vi "Accel2Pos_RatePoints.vi"(8 "Points":u32, 9 "Rate (hz)":dbl, 10 "Start (s)":dbl, 11 "Accel":T1(array[cluster])=[{"A"=5.0, "B"=11.107207345395915, "Start"=0.3585786437626905, "End"=0.6414213562373094, "Center"=0.5, "Velocity"=0.0, "Position"=0.7071067811865475}, {"A"=-5.0, "B"=5.553603672697958, "Start"=1.631370849898476, "End"=2.197056274847714, "Center"=1.914213562373095, "Velocity"=0.7071067811865475, "Position"=-0.7071067811865475}, {"A"=5.0, "B"=11.107207345395915, "Start"=3.18700576850888, "End"=3.4698484809834995, "Center"=3.32842712474619, "Velocity"=-0.7071067811865475, "Position"=0.0}]) -> (1 "Times":dbl[](array[numeric]), 2 "Velocities":dbl[](array[numeric]), 3 "Positions":dbl[](array[numeric]))   [LabVIEW 2014]
panel:
  out "Position/Velocity":cluster{cluster{dbl, dbl}[]}[](graph)
  out "EndTime":dbl
  out "EndIndex":i32
  out "StartIndex":i32
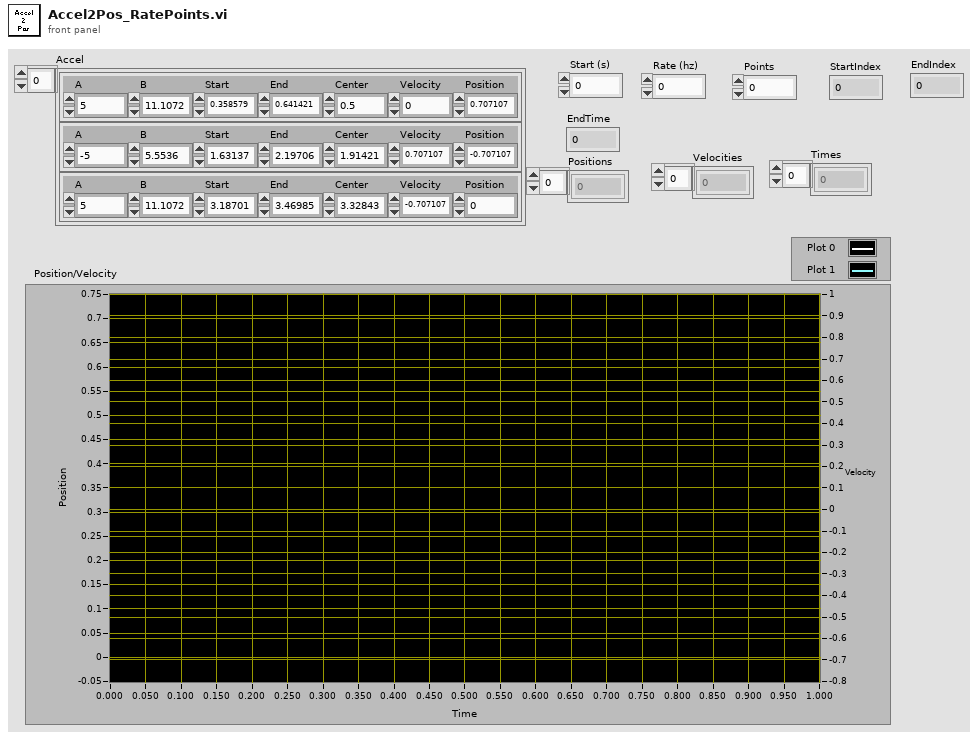
[diagram p1: front panel]
types:
  T1 = cluster{"A":dbl, "B":dbl, "Start":dbl, "End":dbl, "Center":dbl, "Velocity":dbl, "Position":dbl}[]
  T2 = cluster{"A":dbl, "B":dbl, "Start":dbl, "End":dbl, "Center":dbl, "Velocity":dbl, "Position":dbl}
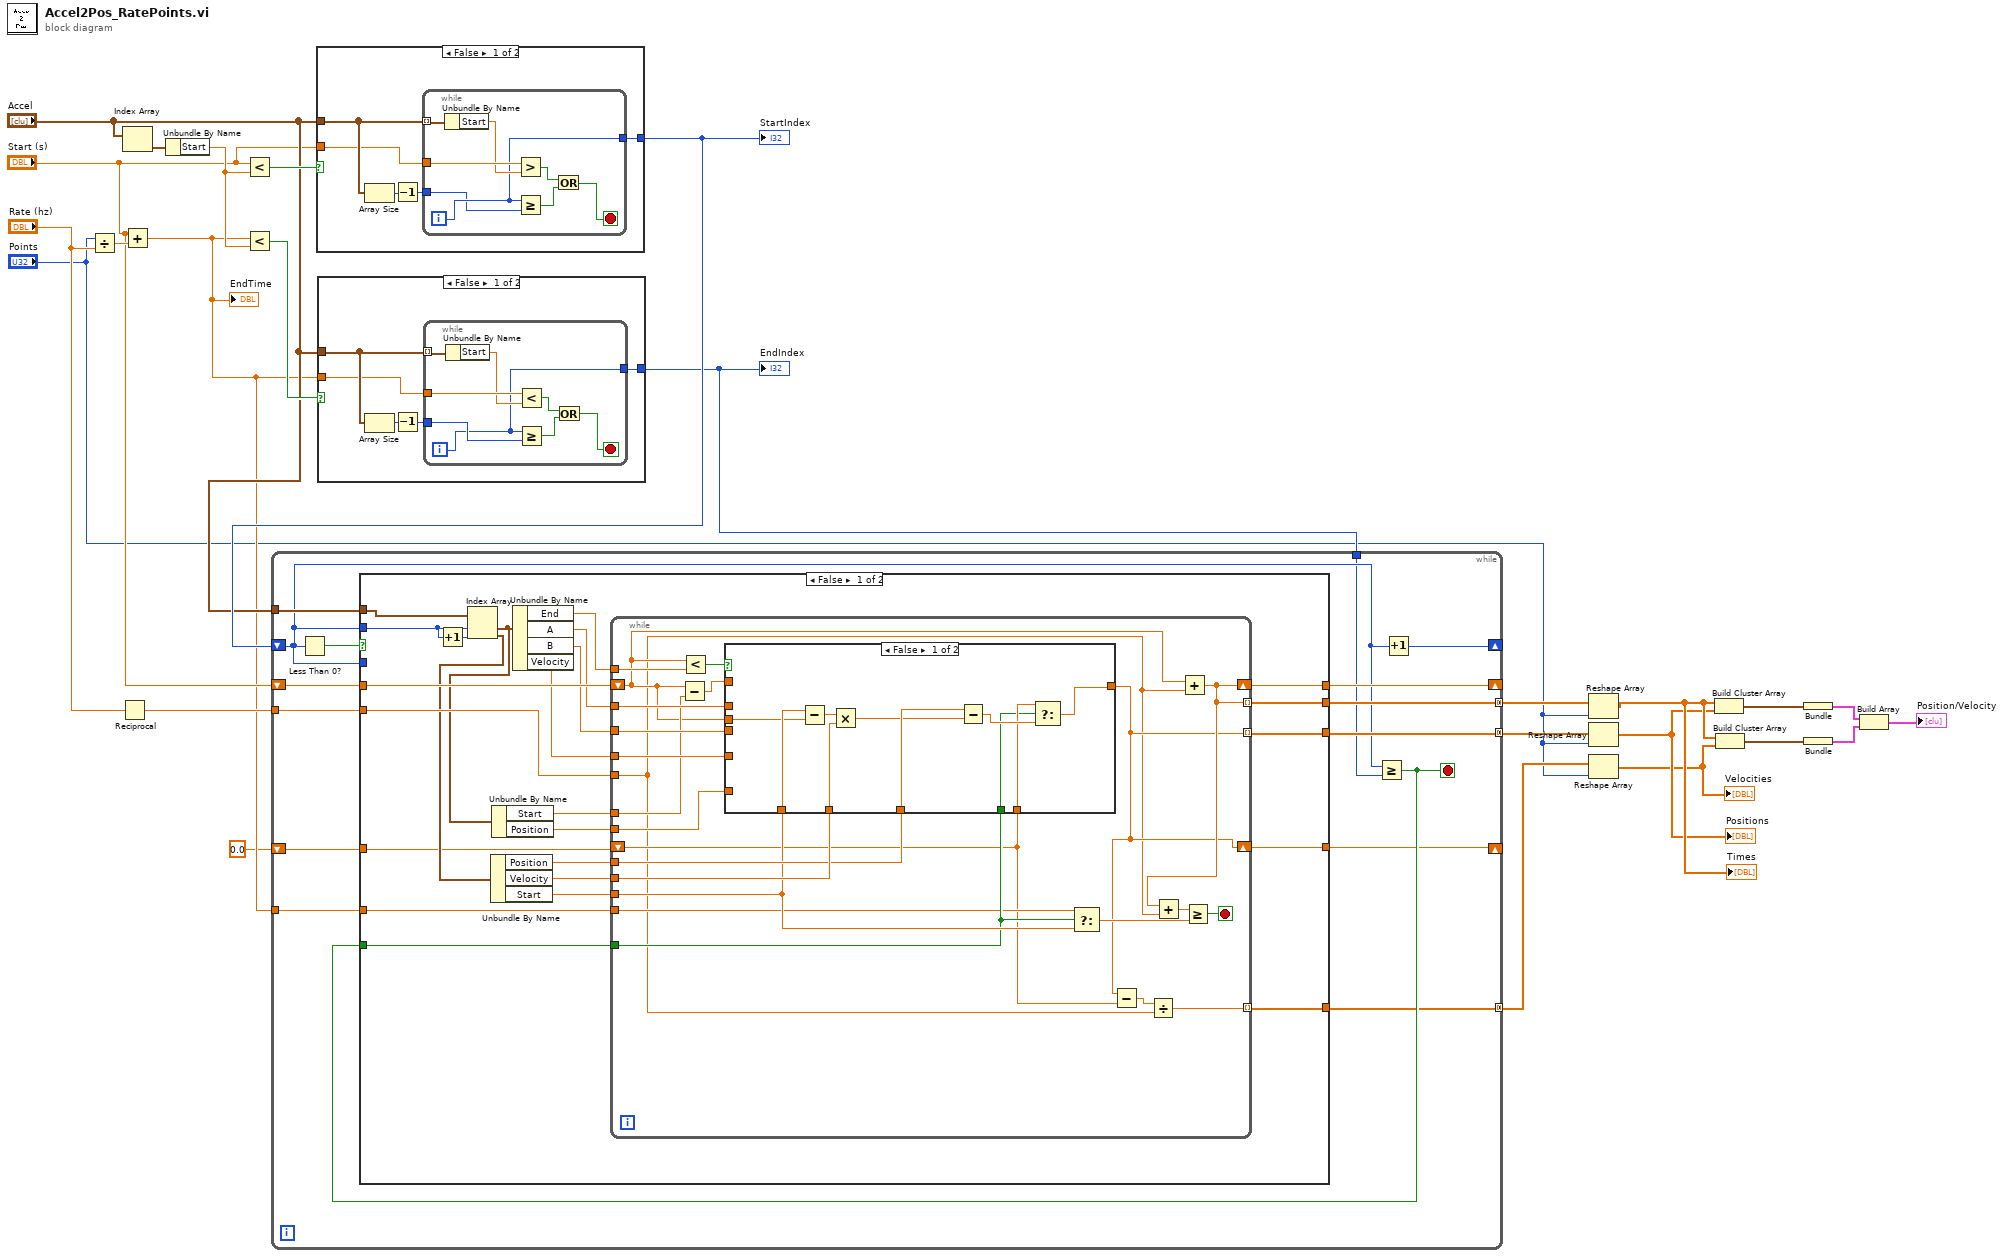
[diagram p0: block diagram]
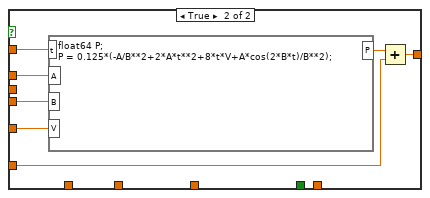
[diagram p2: hidden frame]
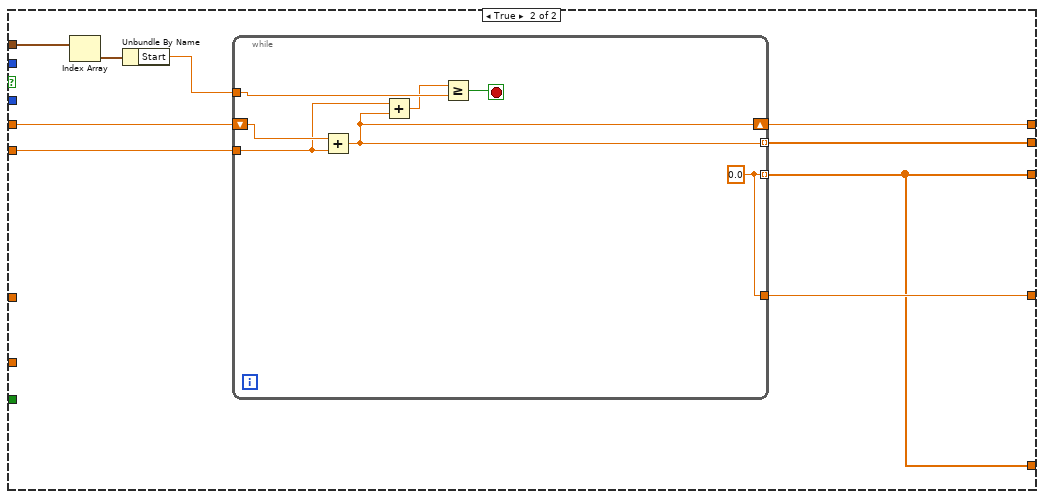
[diagram p3: hidden frame]
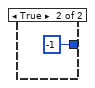
[diagram p4: hidden frame]
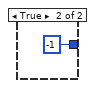
[diagram p5: hidden frame]
diagram:
  n1 = Divide(x="Points", y="Rate (hz)") -> (x/y=w21:dbl)
  n2 = Reciprocal(x="Rate (hz)") -> (1/x=w16:dbl)
  n3 = Index Array(array="Accel") -> (element=w25:T2)  [unwired: 1 in]
  n4 = Add(x="Start (s)", y=w21) -> (x+y=w14:dbl)
  "EndTime" <- w14
  n5 = Unbundle By Name(w25) -> ("Start"=w23:dbl)
  n6 = Less?(x="Start (s)", y=w23) -> (x < y?=w24:bool)
  n7 = Less?(x=w14, y=w23) -> (x < y?=w22:bool)
  n8 = case shown="False" w24 {
    tunnel: [w30 -1] -> w20
    tunnel: "Accel" -> [w29 _]
    tunnel: "Start (s)" -> [w28 _]
    frame False {
      n9 = Array Size(array=w29) -> (size(s)=w27:i32)
      n10 = Decrement(x=w27) -> (x-1=w26:i32)
      n11 = while {
        tunnel: w29 -> [w38] mode=indexing
        tunnel: w28 -> [w37]
        tunnel: [w32] -> w30
        tunnel: w26 -> [w31]
        i -> [w32]
        stop <- w33 stop-if-true
        n12 = Unbundle By Name(w38) -> ("Start"=w36:dbl)
        n13 = Greater?(x=w37, y=w36) -> (0:w35:bool)
        n14 = Greater Or Equal?(x=w32, y=w31) -> (x >= y?=w34:bool)
        n15 = Or(x=w35, y=w34) -> (x .or. y?=w33:bool)
      }
    }
    frame True {
    }
  }
  "StartIndex" <- w20
  n16 = case shown="False" w22 {
    tunnel: [w44 -1] -> w15
    tunnel: "Accel" -> [w43 _]
    tunnel: w14 -> [w42 _]
    frame False {
      n17 = Array Size(array=w43) -> (size(s)=w41:i32)
      n18 = Decrement(x=w41) -> (x-1=w40:i32)
      n19 = while {
        tunnel: w43 -> [w52] mode=indexing
        tunnel: w42 -> [w51]
        tunnel: w40 -> [w49]
        tunnel: [w45] -> w44
        i -> [w45]
        stop <- w46 stop-if-true
        n20 = Unbundle By Name(w52) -> ("Start"=w50:dbl)
        n21 = Less?(x=w51, y=w50) -> (x < y?=w48:bool)
        n22 = Greater Or Equal?(x=w45, y=w49) -> (x >= y?=w47:bool)
        n23 = Or(x=w48, y=w47) -> (x .or. y?=w46:bool)
      }
    }
    frame True {
    }
  }
  "EndIndex" <- w15
  n24 = while {
    shift-right: [w60] -> _
    shift-left: w20 -> [w59]
    tunnel: "Accel" -> [w65]
    shift-right: [w64] -> _
    shift-left: "Start (s)" -> [w67]
    tunnel: w16 -> [w66]
    tunnel: [w63] -> w7 mode=concatenating
    tunnel: [w62] -> w5 mode=concatenating
    tunnel: w15 -> [w58]
    tunnel: w14 -> [w57]
    shift-right: [w56] -> _
    shift-left: 0.0 -> [w55]
    tunnel: [w54] -> w3 mode=concatenating
    stop <- w61 stop-if-true
    n25 = Less Than 0?(x=w59) -> (x < 0?=w68:bool)
    n26 = Greater Or Equal?(x=w59, y=w58) -> (x >= y?=w61:bool)
    n27 = case shown="False" w68 {
      tunnel: w67 -> [w90 w139]
      tunnel: w66 -> [w89 w138]
      tunnel: w65 -> [w92 w141]
      tunnel: [w88 w136] -> w64
      tunnel: [w87 w135] -> w63
      tunnel: [w86 w133] -> w62
      tunnel: w59 -> [_ _]
      tunnel: w61 -> [w73 _]
      tunnel: w59 -> [w91 _]
      tunnel: w57 -> [w72 _]
      tunnel: [w71 w134] -> w56
      tunnel: w55 -> [w70 _]
      tunnel: [w69 w133] -> w54
      frame False {
        n28 = Increment(x=w91) -> (x+1=w85:i32)
        n29 = Index Array(array=w92, index #1=w91, index #2=w85) -> (element #1=w80:T2, element #2=w78:T2)
        n30 = Unbundle By Name(w78) -> ("Position"=w75:dbl, "Velocity"=w76:dbl, "Start"=w77:dbl)
        n31 = Unbundle By Name(w80) -> ("Start"=w74:dbl, "Position"=w79:dbl)
        n32 = Unbundle By Name(w80) -> ("End"=w81:dbl, "A"=w84:dbl, "B"=w83:dbl, "Velocity"=w82:dbl)
        n33 = while {
          tunnel: w84 -> [w106]
          tunnel: w83 -> [w115]
          tunnel: w82 -> [w114]
          shift-right: [w109] -> w88
          shift-left: w90 -> [w103]
          tunnel: w89 -> [w94]
          tunnel: w81 -> [w112]
          tunnel: [w109] -> w87 mode=indexing
          tunnel: w79 -> [w102]
          tunnel: [w97] -> w86 mode=indexing
          tunnel: w77 -> [w101]
          tunnel: w76 -> [w111]
          tunnel: w75 -> [w110]
          tunnel: w74 -> [w105]
          tunnel: w73 -> [w99]
          tunnel: w72 -> [w98]
          shift-right: [w97] -> w71
          shift-left: w70 -> [w96]
          tunnel: [w93] -> w69 mode=indexing
          stop <- w107 stop-if-true
          n34 = Subtract(x=w103, y=w105) -> (x-y=w104:dbl)
          n35 = Less?(x=w103, y=w112) -> (x < y?=w113:bool)
          n36 = case shown="False" w113 {
            tunnel: w106 -> [_ w132]
            tunnel: w115 -> [_ w131]
            tunnel: w114 -> [_ w130]
            tunnel: w104 -> [_ w129]
            tunnel: [w118 w127] -> w97
            tunnel: w101 -> [w125 _]
            tunnel: w111 -> [w123 _]
            tunnel: w110 -> [w122 _]
            tunnel: w103 -> [w120 _]
            tunnel: w102 -> [_ w126]
            tunnel: w96 -> [w117 _]
            tunnel: w99 -> [w116 _]
            frame False {
              n37 = Subtract(x=w125, y=w120) -> (x-y=w124:dbl)
              n38 = Multiply(x=w124, y=w123) -> (x*y=w121:dbl)
              n39 = Subtract(x=w122, y=w121) -> (x-y=w119:dbl)
              n40 = Select(t=w117, s=w116, f=w119) -> (s? t:f=w118:dbl)
            }
            frame True {
              n41 = formula code="float64 P;\nP = 0.125*(-A/B**2+2*A*t**2+8*t*V+A*cos(2*B*t)/B**2);"("A"=w132, "B"=w131, "V"=w130, "t"=w129) -> ("P"=w128:dbl)
              n42 = Add(x=w128, y=w126) -> (x+y=w127:dbl)
            }
          }
          n43 = Select(t=w98, s=w99, f=w101) -> (s? t:f=w100:dbl)
          n44 = Subtract(x=w97, y=w96) -> (x-y=w95:dbl)
          n45 = Divide(x=w95, y=w94) -> (x/y=w93:dbl)
          n46 = Add(x=w103, y=w94) -> (x+y=w109:dbl)
          n47 = Add(x=w109, y=w94) -> (x+y=w108:dbl)
          n48 = Greater Or Equal?(x=w108, y=w100) -> (x >= y?=w107:bool)
        }
      }
      frame True {
        n49 = Index Array(array=w141) -> (element=w140:T2)  [unwired: 1 in]
        n50 = Unbundle By Name(w140) -> ("Start"=w137:dbl)
        n51 = while {
          shift-right: [w144] -> w136
          shift-left: w139 -> [w148]
          tunnel: w138 -> [w145]
          tunnel: w137 -> [w147]
          tunnel: [w144] -> w135 mode=indexing
          tunnel: [w142] -> w133 mode=indexing
          tunnel: [w142] -> w134
          stop <- w146 stop-if-true
          w142 = 0.0
          n52 = Add(x=w148, y=w145) -> (x+y=w144:dbl)
          n53 = Add(x=w145, y=w144) -> (x+y=w143:dbl)
          n54 = Greater Or Equal?(x=w143, y=w147) -> (x >= y?=w146:bool)
        }
      }
    }
    n55 = Increment(x=w59) -> (x+1=w60:i32)
  }
  n56 = Reshape Array(w7, "Points") -> (w6:dbl[])
  "Times" <- w6
  n57 = Reshape Array(w5, "Points") -> (w4:dbl[])
  "Positions" <- w4
  n58 = Reshape Array(w3, "Points") -> (w1:dbl[])
  "Velocities" <- w1
  n59 = Build Cluster Array(w6, w4) -> (w12:cluster{dbl, dbl}[])
  n60 = Build Cluster Array(w6, w1) -> (w11:cluster{dbl, dbl}[])
  n61 = Bundle(w12) -> (w10:cluster{cluster{dbl, dbl}[]})  [unwired: 1 in]
  n62 = Bundle(w11) -> (w9:cluster{cluster{dbl, dbl}[]})  [unwired: 1 in]
  n63 = Build Array(w10, w9) -> (→"Position/Velocity":cluster{cluster{dbl, dbl}[]}[])
